vi "GlobalSender.vi"() -> ()   [LabVIEW 2015]
panel:
  out "headlights":bool
  out "rightdoor":bool
  out "leftdoor":bool
  out "engine stop":bool
  out "engine start":bool
  out "right":bool
  out "left":bool
  out "direction":bool
  out "BRAKES":bool
  out "GAS":bool
  in  "String":string
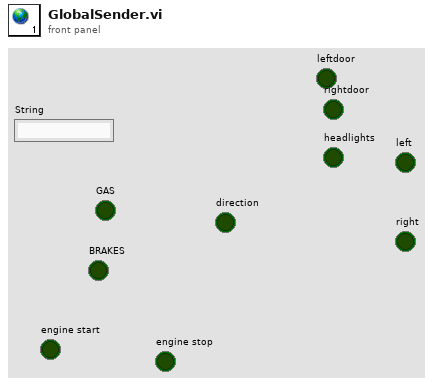
[diagram p1: front panel]
diagram:
